vi "Set Duty Cycle N Chans.vi"(8 "Error In":errorcluster, 9 "Duty Cycles":dbl[](array[numeric]), 10 "PWM Channels":u8[](array[numeric]), 11 "LINX Resource":T1) -> (0 "Error Out":errorcluster, 3 "LINX Resource":T1)   [LabVIEW 2011, in "LMH-LINX.lvlib"]
doc: "Set the duty cycle of the specified PWM channels. \n\nA duty cycle of 0 coresponds to 0% on\nA duty cycle of .33 coresponds to 33% on\nA duty cycle of 1 coresponds to 100% on\netc"
uses:
  LMH-LINX.lvlib
  Private/Type Defs/LINX Ref.ctl
  Private/Type Defs/Platform.ctl
  Private/Type Defs/Interface.ctl
  Private/Device/Type Defs/LINX Device Config.ctl
  Private/Device/Type Defs/TCP Config.ctl
  Private/Device/Type Defs/Channels.ctl
  Private/Type Defs/Peripheral.ctl
  Private/Device/Device.lvlib
  Private/myRIO/myRIO.lvlib
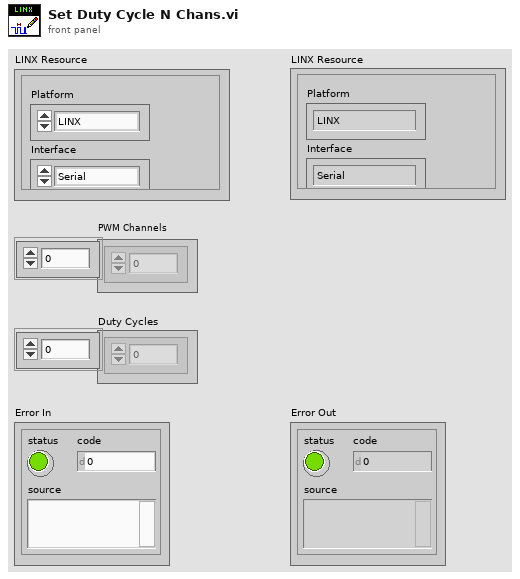
[diagram p1: front panel]
types:
  T1 = typedef "LMH-LINX.lvlib/LINX Ref.ctl" = cluster{"Platform":T2, "Interface":T3, "LINX Device Config":T4}
  T2 = typedef "LMH-LINX.lvlib/Platform.ctl" = enum16{"LINX", "myRIO"}
  T3 = typedef "LMH-LINX.lvlib/Interface.ctl" = enum16{"Serial", "TCP"}
  T4 = typedef "LMH-LINX.lvlib/Device.lvlib/LINX Device Config.ctl" = cluster{"Interface":T3, "COM Port":refnum<visa-resource-name>, "TCP Configuration":T5, "Device Family":u8, "Device ID":u8, "Device Name":string, "TCP Ref":refnum<k5>, "Channels":T6}
  T5 = typedef "LMH-LINX.lvlib/Device.lvlib/TCP Config.ctl" = cluster{"IP Address":string, "Port":u16}
  T6 = typedef "LMH-LINX.lvlib/Channels.ctl" = cluster{"DI":u8[], "DO":u8[], "AI":u8[], "AO":u8[], "PWM":u8[], "QE":u8[], "UART":u8[], "I2C 2":u8[], "SPI":u8[], "CAN":u8[], "Servo":u8[], "AI Ref (V)":dbl, "AO Ref (V)":dbl, "AO Resolution (Bits)":u8}
  T7 = typedef "LMH-LINX.lvlib/Peripheral.ctl" = enum8{"DI", "DO", "AI", "AO", "PWM", "QE", "UART", "I2C", "SPI", "CAN", "Servo"}
  T8 = typedef "PWM.lvlib/PWM Reference.ctl" = cluster{"myRIO Reference":T9, "PWM Channels Enum":T13, "PWM Configuration":T14}
  T9 = typedef "myRIO Generic Hardware Reference.ctl" = cluster{"myRIO Model":T10, "myRIO Hardware Reference":T11}
  T10 = typedef "Hardware Version Enum.ctl" = enum16{"Unknown", "myRIO-1900", "myRIO-1950"}
  T11 = typedef "myRIO v1.0 Reference.ctl" = cluster{"Generic FPGA Reference":T12, "Allow multiple opens":bool}
  T12 = typedef "Generic FPGA Reference.ctl" = refnum<k20>
  T13 = typedef "PWM Channels Enum.ctl" = enum16{"Not Connected", "C/PWM0", "C/PWM1", "A/PWM0", "A/PWM1", "A/PWM2", "B/PWM0", "B/PWM1", "B/PWM2"}
  T14 = typedef "PWM.lvlib/PWM Configuration.ctl" = cluster{"Frequency":dbl, "Duty Cycle":dbl}
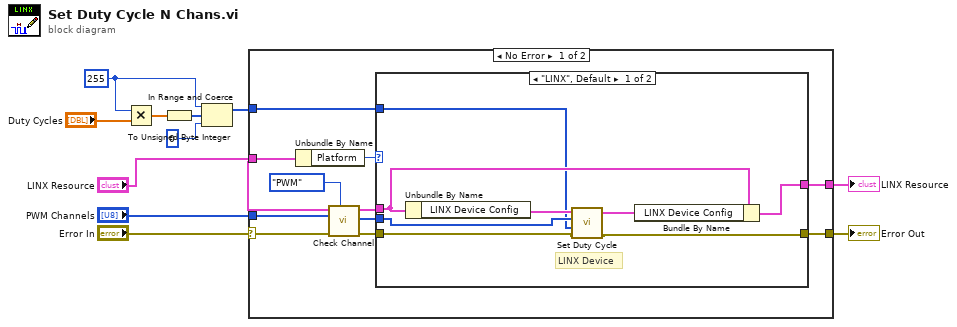
[diagram p0: block diagram]
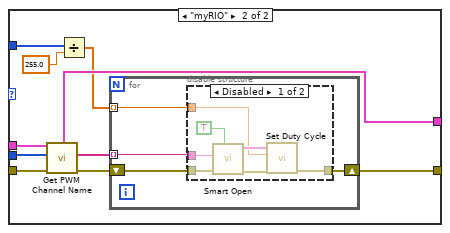
[diagram p2: hidden frame]
diagram:
  w5 = u8 255
  n1 = Multiply(x=w5, y="Duty Cycles") -> (x*y=w4:dbl[])
  n2 = To Unsigned Byte Integer(number=w4) -> (unsigned 8bit integer=w3:u8[])
  n3 = In Range and Coerce(upper limit=w5, x=w3, lower limit=u8 0) -> (coerced(x)=w1:u8[])  [unwired: 1 out]
  n4 = case shown="No Error" "Error In" {
    selector: "Error In" -> [w12 w53]
    tunnel: [w21 w53] -> w11
    tunnel: [w20 w52] -> w10
    tunnel: "LINX Resource" -> [w18 w52]
    tunnel: w1 -> [w14 _]
    tunnel: "PWM Channels" -> [w13 _]
    frame No Error {
      n5 = Unbundle By Name(w18) -> ("Platform"=w22:T2)
      n6 = call "Check Channel.vi"("Peripheral"=Peripheral."PWM", "Error In"=w12, "Channels"=w13, "LINX Resource"=w18) -> ("Error Out"=w16:errorcluster, "Channels"=w15:u8[], "LINX Resource"=w17:T1)  [unwired: 5 in]
      n7 = case shown="\"LINX\", Default" w22 {
        tunnel: w16 -> [w27 w38]
        tunnel: w17 -> [w30 w39]
        tunnel: [w28 w35] -> w21
        tunnel: [w29 w39] -> w20
        tunnel: w14 -> [w23 w33]
        tunnel: w15 -> [w24 w37]
        frame "LINX", Default {
          # "LINX Device"
          n8 = Unbundle By Name(w30) -> ("LINX Device Config"=w25:T4)
          n9 = call <vilib>:"Set Duty Cycle.vi"("Error In"=w27, "Duty Cycles (0-255)"=w23, "Channels"=w24, "LINX Device Config"=w25) -> ("Error Out"=w28:errorcluster, "LINX Device Config"=w26:T4)  [unwired: 6 in]
          n10 = Bundle By Name(cluster=w30, "LINX Device Config"=w26) -> (w29:T1)
        }
        frame "myRIO" {
          n11 = call "Get PWM Channel Name.vi"("Error In"=w38, "PWM Channel Nums"=w37) -> ("Error Out"=w36:errorcluster, "PWM Channels"=w34:string[])  [unwired: 8 in]
          n12 = Divide(x=w33, y=255.0) -> (x/y=w31:dbl[])
          n13 = for {
            shift-right: [w43] -> w35
            shift-left: w36 -> [w42]
            tunnel: w34 -> [w41] mode=indexing
            tunnel: w31 -> [w40] mode=indexing
            n14 = disable-structure shown="Disabled" {
              disable-tunnel: [w47 w51] -> w43
              disable-tunnel: w42 -> [w46 w51]
              disable-tunnel: w41 -> [w45 _]
              disable-tunnel: w40 -> [w44 _]
              frame Disabled {
                n15 = call <vilib>:"Smart Open.vi"("Allow multiple opens?"=TRUE, "error in (no error)"=w46, "Channel Name"=w45) -> ("error out"=w50:errorcluster, "PWM Ref Out"=w49:T8)  [unwired: 7 in]
                n16 = call <vilib>:"Set Duty Cycle.vi"("error in (no error)"=w50, "Duty Cycle (0-1)"=w44, "PWM Ref In"=w49) -> ("error out"=w47:errorcluster)  [unwired: 6 in, 1 out]
              }
              frame Enabled {
              }
            }
          }
        }
      }
    }
    frame Error {
    }
  }
  "Error Out" <- w11
  "LINX Resource" <- w10
